vi "Redis@Transaction__Parameter.vi"(1 "ParamterIn":string) -> (0 "ParamterOut":string)   [LabVIEW 2020]
panel:
  in  "Message=":string
  in  "TimeOut=":string(combo)
  in  "Variable=":string(combo)
  in  "Section":string(combo)
  in  "CMD":string
  in  "RedisSession":string(combo)
  in  "Confirm":bool
  # "RedisSession(,Variable=,TimeOut=XXX, Message=XXX) \nCMD"
  # "@"
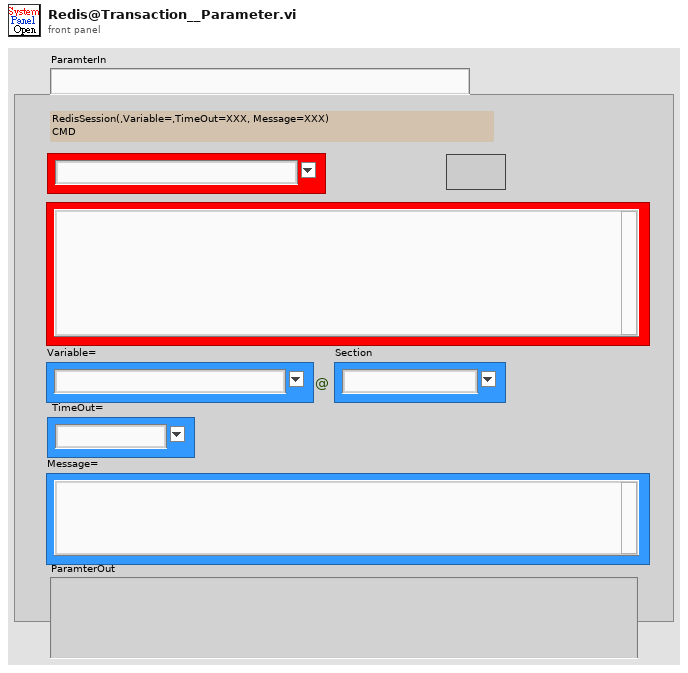
[diagram p1: front panel]
types:
  T1 = enum16{"Get", "Init", "Set", "Delete", "GetElement", "Inc", "Dec"}
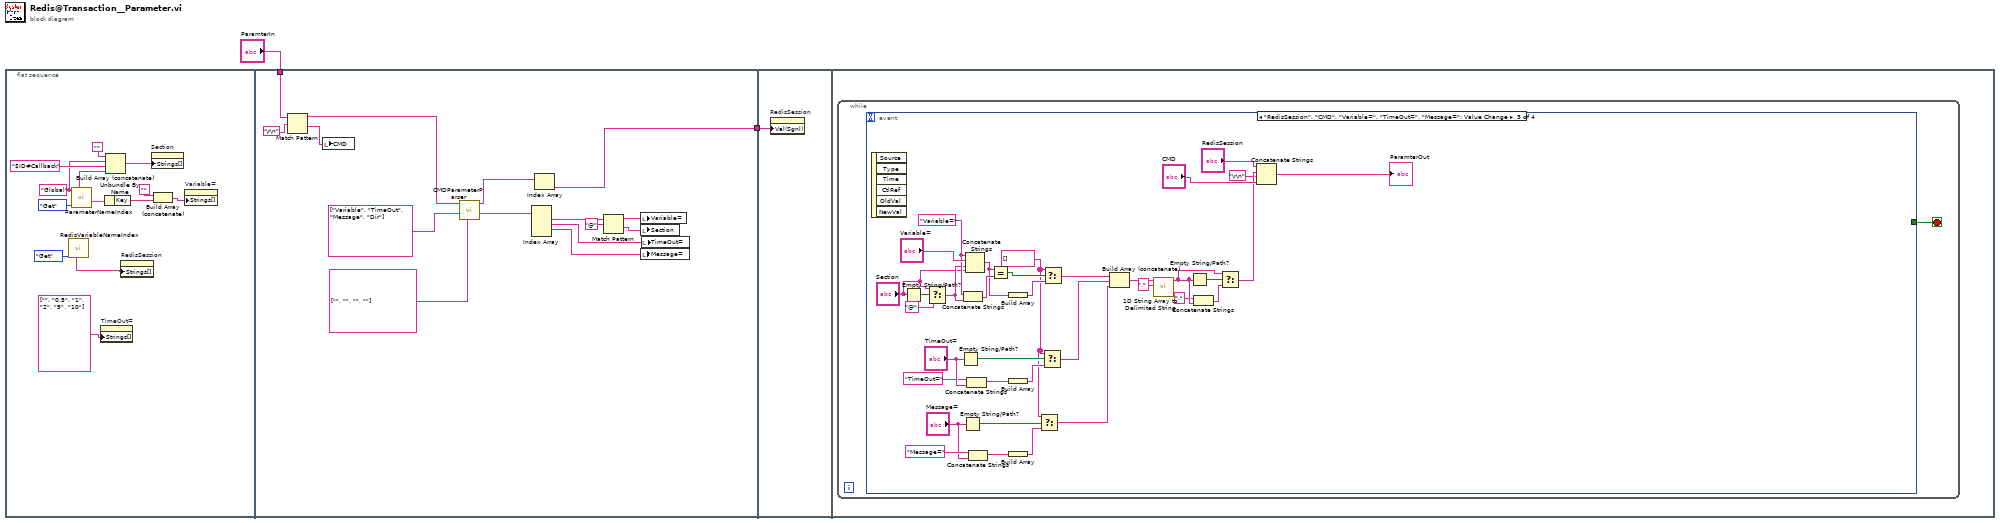
[diagram p0: block diagram]
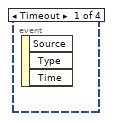
[diagram p2: hidden frame]
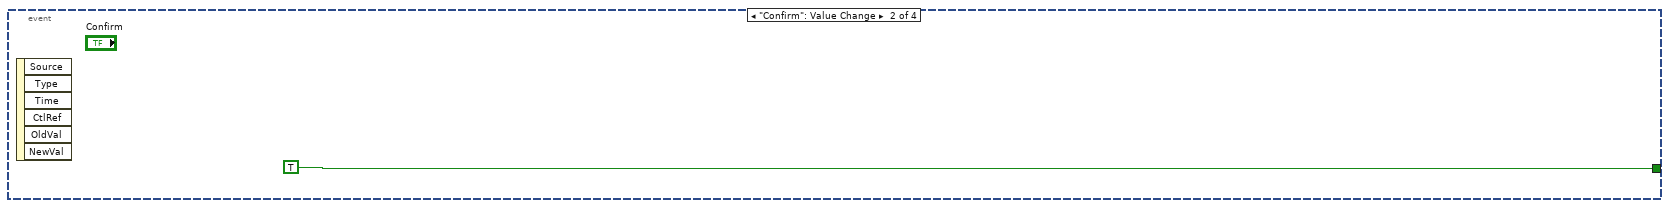
[diagram p3: hidden frame]
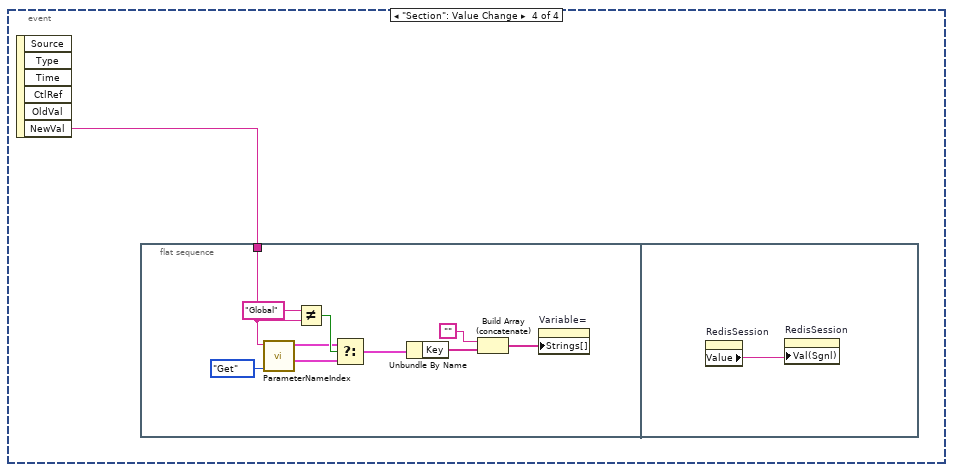
[diagram p4: hidden frame]
diagram:
  n1 = flat-sequence {
    tunnel: "ParamterIn" -> [w19]
    tunnel: [w27] -> w1
    tunnel: w1 -> [w31]
    frame #0 {
      w6 = "Global" ("VariableSection")
      n2 = call "RedisVariableNameIndex.vi"("OP"=enum16{"Add", "Init", "Get"}."Get") -> ("RedisSessionS"=w8:string[])  [unwired: 6 in, 4 out]
      n3 = call "ParameterNameIndex.vi"("OP"=T1."Get", "VariableSection"=w6) -> ("GlobalKeyValue"=w7:cluster{"Key":string[], "Value":string[]}, "SectionList"=w14:string[])  [unwired: 3 in, 5 out]
      n4 = property on="TimeOut=" class="CmbBox"("Strings[]"=string[] ["", "0.5", "1", "2", "5", "10"] ("Strings []")) -> ()  [unwired: 2 in, 2 out]
      n5 = Unbundle By Name(w7) -> ("Key"=w4:string[])
      n6 = Build Array (concatenate)("", w6, "$ID#Callback" ("VariableSection"), w14) -> (w13:string[])
      n7 = property on="RedisSession" class="CmbBox"("Strings[]"=w8) -> ()  [unwired: 2 in, 2 out]
      n8 = property on="Section" class="CmbBox"("Strings[]"=w13) -> ()  [unwired: 2 in, 2 out]
      n9 = Build Array (concatenate)("", w4) -> (w3:string[])
      n10 = property on="Variable=" class="CmbBox"("Strings[]"=w3) -> ()  [unwired: 2 in, 2 out]
    }
    frame #1 {
      n11 = Match Pattern(string=w19, regular expression="\r\n") -> (before substring=w16:string, after substring=w17:string)  [unwired: 1 in, 2 out]
      n12 = local write "CMD"(w17) -> ()
      n13 = call "CMDParameterParser.vi"("DeafultValues"=string[] ["", "", "", ""], "RequiredKeys"=string[] ["Variable", "TimeOut", "Message", "Dir"], "CMDParameter"=w16) -> ("KeyValues"=w26:string[], "Input"=w28:string[])  [unwired: 6 in, 1 out]
      n14 = Index Array(array=w26) -> (element #1=w25:string, element #2=w22:string, element #3=w21:string)  [unwired: 4 in, 1 out]
      n15 = Index Array(array=w28) -> (element=w27:string)  [unwired: 1 in]
      n16 = Match Pattern(string=w25, regular expression="@") -> (before substring=w23:string, after substring=w20:string)  [unwired: 1 in, 2 out]
      n17 = local write "Variable="(w23) -> ()
      n18 = local write "Section"(w20) -> ()
      n19 = local write "Message="(w21) -> ()
      n20 = local write "TimeOut="(w22) -> ()
    }
    frame #2 {
      n21 = property on="RedisSession" class="CmbBox"("Val(Sgnl)"=w31) -> ()  [unwired: 2 in, 2 out]
    }
    frame #3 {
      n22 = while {
        stop <- w32 stop-if-true
        n23 = event shown="[2] \"RedisSession\", \"CMD\", \"Variable=\", \"TimeOut=\", \"Message=\": Value Change" {
          selector: _ -> [_ _ _ _]
          dyn-events: _ -> [_ _ _ _]
          timeout: _ -> [_ _ _ _]
          tunnel: [_ TRUE _ _] -> w32
          event Timeout {
            n24 = event-data() -> ()  [unwired: 1 in, 3 out]
          }
          event "Confirm": Value Change {
            n25 = event-data() -> ()  [unwired: 1 in, 6 out]
          }
          event "RedisSession", "CMD", "Variable=", "TimeOut=", "Message=": Value Change {
            w51 = string[] [] ("t")
            w64 = "Variable=" ("string")
            n26 = event-data() -> ()  [unwired: 1 in, 6 out]
            n27 = Empty String/Path?(string/path="Section") -> (empty?=w40:bool)
            n28 = Select(t="Section", s=w40, f="@") -> (s? t:f=w38:string)
            n29 = Empty String/Path?(string/path="TimeOut=") -> (empty?=w63:bool)
            n30 = Empty String/Path?(string/path="Message=") -> (empty?=w58:bool)
            n31 = Concatenate Strings(w64, w38) -> (w57:string)
            n32 = Concatenate Strings(w64, "Variable=", w38, "Section") -> (w41:string)
            n33 = Concatenate Strings("TimeOut=" ("string"), "TimeOut=") -> (w55:string)
            n34 = Concatenate Strings("Message=" ("string"), "Message=") -> (w53:string)
            n35 = Equal?(x=w41, y=w57) -> (x = y?=w65:bool)
            n36 = Build Array(w41) -> (w56:string[])
            n37 = Build Array(w55) -> (w54:string[])
            n38 = Build Array(w53) -> (w52:string[])
            n39 = Select(t=w51, s=w58, f=w52) -> (s? t:f=w48:string[])
            n40 = Select(t=w51, s=w63, f=w54) -> (s? t:f=w49:string[])
            n41 = Select(t=w51, s=w65, f=w56) -> (s? t:f=w50:string[])
            n42 = Build Array (concatenate)(w50, w49, w48) -> (w47:string[])
            n43 = call <vilib>:"1D String Array to Delimited String.vi"("delimiter"=",", "string array"=w47) -> ("delimited string"=w44:string)  [unwired: 9 in]
            n44 = Empty String/Path?(string/path=w44) -> (empty?=w45:bool)
            n45 = Concatenate Strings("," ("string"), w44) -> (w42:string)
            n46 = Select(t=w44, s=w45, f=w42) -> (s? t:f=w35:string)
            n47 = Concatenate Strings("RedisSession", w35, "\r\n", "CMD") -> (→"ParamterOut":string)
          }
          event "Section": Value Change {
            n48 = event-data() -> ("NewVal"=w69:string)  [unwired: 1 in, 5 out]
            n49 = flat-sequence {
              tunnel: w69 -> [w78]
              frame #0 {
                n50 = call "ParameterNameIndex.vi"("OP"=T1."Get", "VariableSection"=w78) -> ("GlobalKeyValue"=w74:cluster{"Key":string[], "Value":string[]}, "SectionKeyValue"=w75:cluster{"Key":string[], "Value":string[]})  [unwired: 3 in, 5 out]
                n51 = Not Equal?(x="Global", y=w78) -> (x != y?=w76:bool)
                n52 = Select(t=w75, s=w76, f=w74) -> (s? t:f=w73:cluster{"Key":string[], "Value":string[]})
                n53 = Unbundle By Name(w73) -> ("Key"=w72:string[])
                n54 = Build Array (concatenate)("", w72) -> (w70:string[])
                n55 = property on="Variable=" class="CmbBox"("Strings[]"=w70) -> ()  [unwired: 2 in, 2 out]
              }
              frame #1 {
                n56 = property on="RedisSession" class="CmbBox"() -> ("Value"=w80:string)  [unwired: 2 in, 2 out]
                n57 = property on="RedisSession" class="CmbBox"("Val(Sgnl)"=w80) -> ()  [unwired: 2 in, 2 out]
              }
            }
          }
        }
      }
    }
  }
